vi "As Minimal Cluster.vi"(8 "error in (no error)":errorcluster, 11 "Generic Controller in":refnum<class "Generic Plugin.lvclass">) -> (0 "error out":errorcluster, 2 "Minimal Cluster out":T1, 3 "Generic Controller out":refnum<class "Generic Plugin.lvclass">)   [LabVIEW 2020, in "Generic Plugin.lvclass"]
uses:
  Generic Plugin.lvclass
  Minimal Controller Cluster.ctl
  Generic Plugin.lvclass/Generic Plugin.ctl
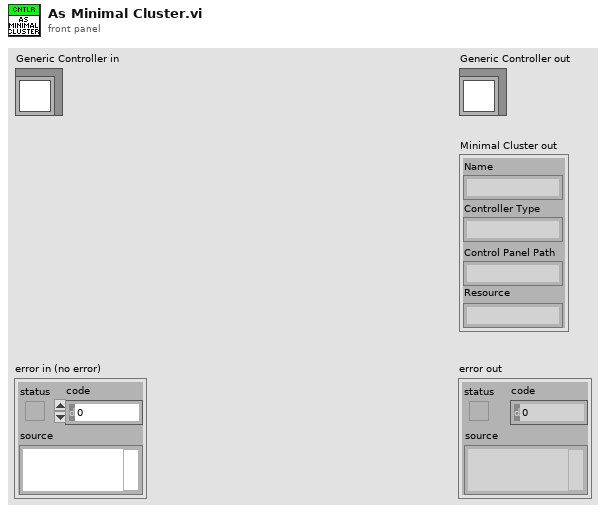
[diagram p1: front panel]
types:
  T1 = typedef "Generic Plugin.lvclass/Minimal Controller Cluster.ctl" = cluster{"Name":string, "Controller Type":string, "Control Panel Path":string, "Resource":string}
  T2 = typedef "Generic Plugin.lvclass/Controller Type.ctl" = enum16{"Invalid", "Temperature Controller", "Pump Controller", "Generic Optimizer", "LC Parser"}
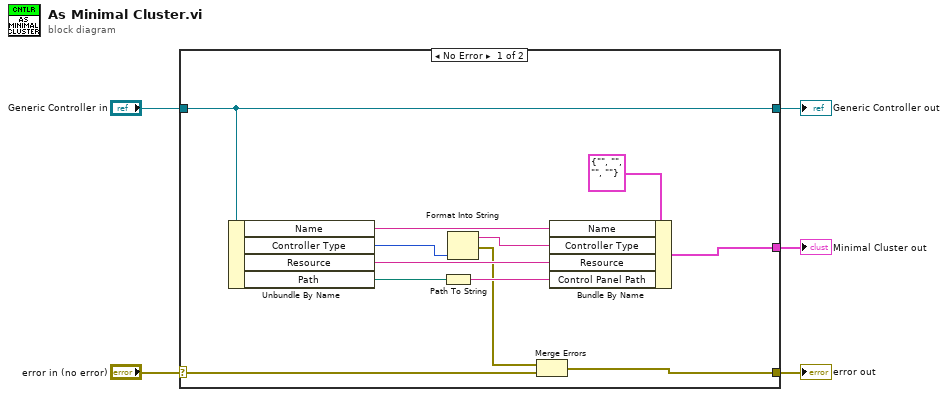
[diagram p0: block diagram]
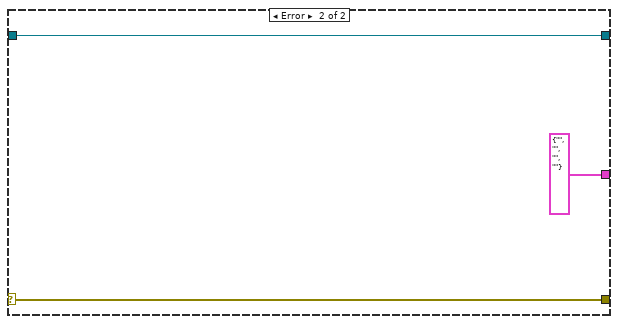
[diagram p2: hidden frame]
diagram:
  n1 = case shown="No Error" "error in (no error)" {
    selector: "error in (no error)" -> [w17 w20]
    tunnel: [w7 w20] -> w4
    tunnel: [w16 w19] -> w2
    tunnel: "Generic Controller in" -> [w16 w19]
    tunnel: [w12 T1 {"Name"="", "Controller Type"="", "Control Panel Path"="", "Resource"=""} ("output cluster")] -> w1
    frame No Error {
      n2 = Unbundle By Name(w16) -> ("Name"=w15:string, "Controller Type"=w11:T2, "Resource"=w14:string, "Path"=w9:path)
      n3 = Path To String(path=w9) -> (string=w8:string)
      n4 = Format Into String(w11) -> (resulting string=w10:string, error out=w6:errorcluster)  [unwired: 3 in]
      n5 = Merge Errors(w6, w17) -> (w7:errorcluster)
      n6 = Bundle By Name(cluster=T1 {"Name"="", "Controller Type"="", "Control Panel Path"="", "Resource"=""} ("output cluster"), "Name"=w15, "Controller Type"=w10, "Resource"=w14, "Control Panel Path"=w8) -> (w12:T1)
    }
    frame Error {
    }
  }
  "error out" <- w4
  "Generic Controller out" <- w2
  "Minimal Cluster out" <- w1
